vi "Sub Panel Test.vi"() -> ()   [LabVIEW 2017]
uses:
  Development Tools/Mini Explorer/Source/Item Tree/ID to Tree Items/Tree Item Type.ctl
  Development Tools/Mini Explorer/Source/DSF Mini Explorer.vi
  DSF Core.lvlibp/Classes/Configuration/Configuration Session.lvclass
  Development Tools/Mini Explorer/DSF Mini Explorer.lvlib
panel:
  in  "dsf configuration file path":path=path "C:/Users/Admin/Desktop/test.dsf"
  in  "stop":bool
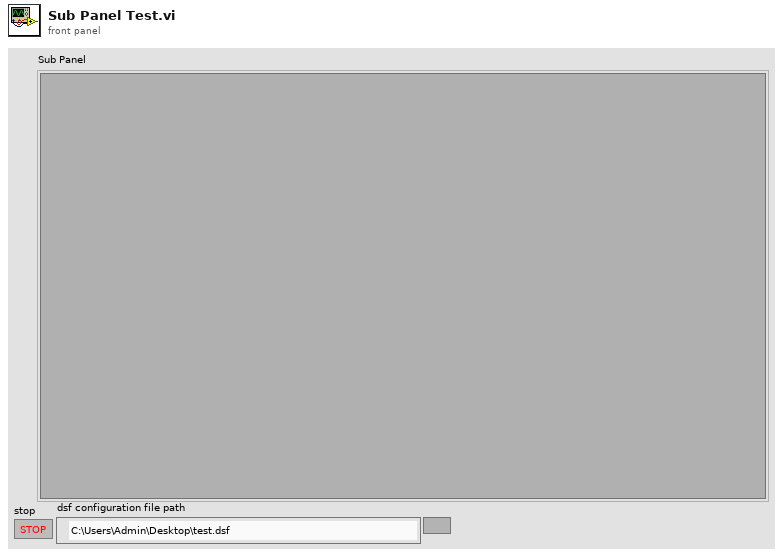
[diagram p1: front panel]
types:
  T1 = typedef "DSF Mini Explorer.lvlib/Tree Item Type.ctl" = enum16{"Plugin", "Group", "Transfer", "Channel", "Setting"}
  T2 = typedef "DSF Mini Explorer.lvlib/Application Data.ctl" = cluster{"Item Tree Control":refnum<vi>, "Value Tree Control":refnum<vi>, "DSF Refnum":refnum<class "Configuration Session.lvclass">, "Top-Level VI":refnum<vi>, "View State":T3}
  T3 = typedef "DSF Mini Explorer.lvlib/View Mode.ctl" = enum16{"Tree", "List"}
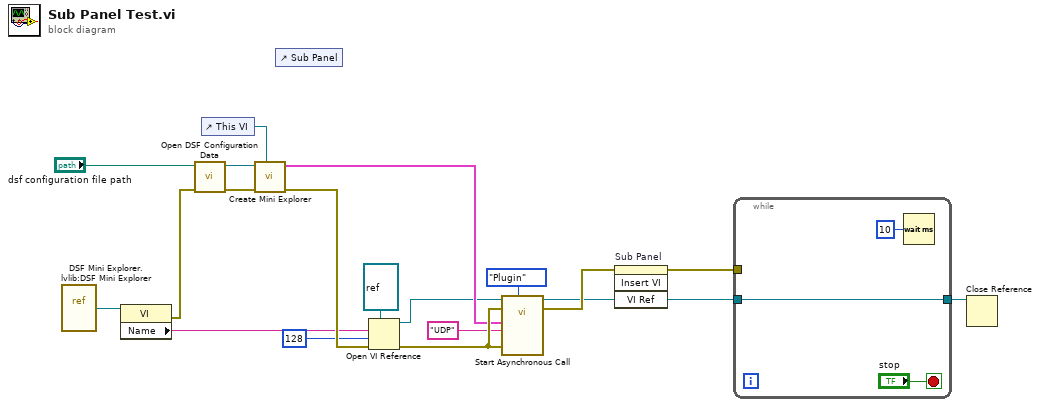
[diagram p0: block diagram]
diagram:
  n1 = vi-ref "DSF Mini Explorer.lvlib:DSF Mini Explorer.vi"() -> (w15:refnum<vi>)
  n2 = property class="VI"(reference=w15) -> (error out=w2:errorcluster, "Name"=w14:string)  [unwired: 1 in, 1 out]
  n3 = call "Open DSF Configuration Data.vi"("error in (no error)"=w2, "dsf configuration file path"="dsf configuration file path") -> ("error out"=w17:errorcluster, "Configuration Session"=w16:refnum<class "Configuration Session.lvclass">)  [unwired: 5 in, 3 out]
  n4 = control-ref of="This VI"() -> (w9:refnum<vi>)
  n5 = call "Create Mini Explorer.vi"("Top-Level VI"=w9, "error in (no error)"=w17, "DSF Confguration Session"=w16) -> ("error out"=w18:errorcluster, "explorer data"=w7:T2)  [unwired: 7 in]
  n6 = control-ref of="Sub Panel"() -> ()  [unwired: 1 out]
  n7 = Open VI Reference(type specifier VI Refnum (for type only)=refnum<vi> refnum, vi path=w14, options=128, error in (no error)=w18) -> (vi reference=w6:refnum<vi>, error out=w19:errorcluster)  [unwired: 2 in]
  n8 = call-by-ref "Start Asynchronous Call"(reference=w6, error in=w19, "Item Type"=Tree_Item_Type."Plugin", 8:"error in (no error)"=w19, "Item ID"="UDP", "explorer data"=w7) -> (reference out=w3:refnum<vi>, error out=w5:errorcluster)  [unwired: 7 in, 1 out]
  n9 = invoke on="Sub Panel" class="SubPnl" method="Insert VI"(error in=w5, "VI Ref"=w3) -> (error out=w4:errorcluster)  [unwired: 2 in, 3 out]
  n10 = while {
    tunnel: w3 -> [w20]
    tunnel: [w20] -> w10
    tunnel: w4 -> [_]
    stop <- "stop" stop-if-true
    n11 = Wait (ms)(milliseconds to wait=u32 10) -> ()  [unwired: 1 out]
  }
  n12 = Close Reference(reference=w10) -> ()  [unwired: 1 in, 1 out]
